vi "AlGaInPAs_v21a.vi"(2 "Debug Mode":bool, 3 "Elapsed Time(s)":dbl, 4 "State":enum16{"Edit", "Start", "Run", "End", "Idle"}(ring), 5 "Argument List In":string[](array[string])) -> (0 "Status Out":string, 1 "Argument List Out":string[](array[string]))   [LabVIEW 2011]
uses:
  high_level_proc/source_noDilute.ctl
  high_level_proc/source_noDilution.ctl
panel:
  in  "Zn bubbler":T1={"Dilution"=FALSE, "Calculated"=0, "MFC1 flow"=0.0, "MFC2 flow"=10.0, "MFC3 flow"=100.0, "Bubbler (main)"={"Flow"=0.0, "Prep"=FALSE, "Run"=FALSE, "Active"=FALSE}} caption="Al" {"Bubbler (main)"."Flow" format="%.2f"; "MFC1 flow" format="%.4f"; "MFC3 flow" format="%.1f"; "MFC2 flow" format="%.2f"; "Calculated" items=["Flow", "MFC1", "MFC2", "MFC3"]}
  in  "Array":refnum<vi>[](array[refnum])
  in  "Al bubbler":T2 caption="Al" {"Flow" format="%.2f"}
  in  "Se bubbler":T1={"Dilution"=FALSE, "Calculated"=0, "MFC1 flow"=0.0, "MFC2 flow"=10.0, "MFC3 flow"=100.0, "Bubbler (main)"={"Flow"=0.0, "Prep"=FALSE, "Run"=FALSE, "Active"=FALSE}} caption="Al" {"Bubbler (main)"."Flow" format="%.2f"; "MFC1 flow" format="%.4f"; "MFC3 flow" format="%.1f"; "MFC2 flow" format="%.2f"; "Calculated" items=["Flow", "MFC1", "MFC2", "MFC3"]}
  in  "P bubbler":T2 caption="Al" {"Flow" format="%.2f"}
  in  "As gas":T2 caption="Al" {"Flow" format="%.2f"}
  in  "P gas":T2 caption="Al" {"Flow" format="%.2f"}
  in  "In bubbler":T2 caption="Al" {"Flow" format="%.2f"}
  in  "Tab Control":T3(tab)
  out "Al Prep":bool caption="Pre-run"
  out "Al Run":bool caption="Run"
  out "Al Flow":dbl caption="Al Flow (0-100 sscm)" format="%.2f"
  out "Ga MFC1 flow":dbl caption="R1 (0-10 sscm)" format="%.4f"
  out "Ga MFC3 flow":dbl=100.0 caption="R3 (0-1000 sscm)" format="%.1f"
  out "Ga MFC2 flow":dbl=10.0 caption="R2 (0-100 sscm)" format="%.2f"
  out "Ga Calculated":u16(ring)=1 caption="Calculated" items=["Ga flow", "MFC1", "MFC2", "MFC3"]
  out "Ga Dilution":bool caption="Dilute"
  out "Ga Prep":bool caption="Pre-run"
  out "Ga Run":bool caption="Run"
  out "Ga Flow":dbl caption="Ga Flow (0-10 sscm)" format="%.2f"
  out "In Prep":bool caption="Pre-run"
  out "In Run":bool caption="Run"
  out "In Flow":dbl caption="In Flow (0-100 sscm)" format="%.2f"
  out "P gas Run":bool caption="Run"
  out "P gas Prep":bool caption="Pre-run"
  out "P gas Flow":dbl caption="PH3 Flow (0-100 sscm)" format="%.2f"
  out "As gas Prep":bool caption="Pre-run"
  out "As gas Run":bool caption="Run"
  out "As gas Flow":dbl caption="AsH3 Flow (0-10 sscm)" format="%.2f"
  out "P liq Prep":bool caption="Pre-run"
  out "P liq Run":bool caption="Run"
  out "P liq Flow":dbl caption="P bubbler Flow (0-100 sscm)" format="%.2f"
  out "Zn Flow":dbl caption="Zn Flow (0-10 sscm)" format="%.2f"
  out "Zn Run":bool caption="Run"
  out "Zn Prep":bool caption="Pre-run"
  out "Zn  Dilution":bool caption="Dilute"
  out "Zn Calculated":u16(ring)=1 caption="Calculated" items=["Ga flow", "MFC1", "MFC2", "MFC3"]
  out "Zn MFC2 flow":dbl=10.0 caption="R2 (0-100 sscm)" format="%.2f"
  out "Zn MFC3 flow":dbl=100.0 caption="R3 (0-1000 sscm)" format="%.1f"
  out "Zn MFC1 flow":dbl caption="R1 (0-10 sscm)" format="%.4f"
  out "Se MFC1 flow":dbl caption="R1 (0-10 sscm)" format="%.4f"
  out "Se MFC3 flow":dbl=100.0 caption="R3 (0-1000 sscm)" format="%.1f"
  out "Se MFC2 flow":dbl=10.0 caption="R2 (0-100 sscm)" format="%.2f"
  out "Se Calculated":u16(ring)=1 caption="Calculated" items=["Ga flow", "MFC1", "MFC2", "MFC3"]
  out "Se Dilution":bool caption="Dilute"
  out "Se Prep":bool caption="Pre-run"
  out "Se Run":bool caption="Run"
  out "Se Flow":dbl caption="Se Flow (0-10 sscm)" format="%.2f"
  in  "Ga bubbler":T1={"Dilution"=FALSE, "Calculated"=0, "MFC1 flow"=0.0, "MFC2 flow"=10.0, "MFC3 flow"=100.0, "Bubbler (main)"={"Flow"=0.0, "Prep"=FALSE, "Run"=FALSE, "Active"=FALSE}} caption="Al" {"Bubbler (main)"."Flow" format="%.2f"; "MFC1 flow" format="%.4f"; "MFC3 flow" format="%.1f"; "MFC2 flow" format="%.2f"; "Calculated" items=["Flow", "MFC1", "MFC2", "MFC3"]}
  out "prep_done":bool
  out "run started":bool
  out "first":bool=TRUE
  out "total time":dbl
  out "is OK?":bool
  in  "prep_time":dbl
  in  "Cancel":bool
  in  "OK":bool
  out "tTotal(s) 2":dbl
  # "s"
  # "Add pre-run time to run time in editor."
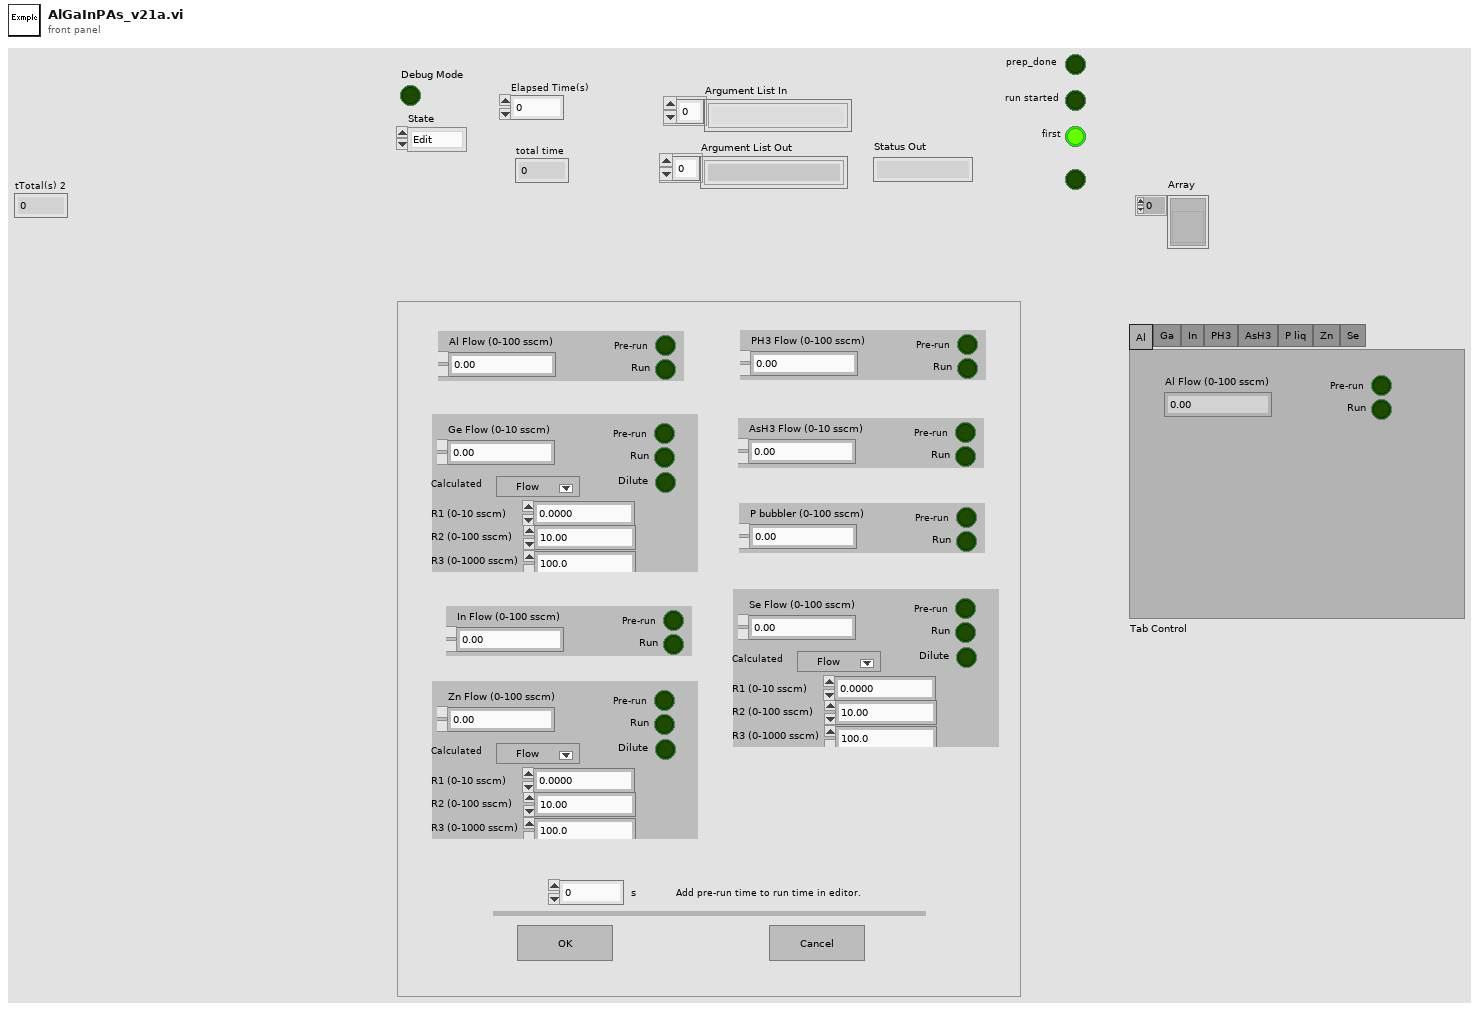
[diagram p1: front panel]
types:
  T1 = typedef "source_noDilute.ctl" = cluster{"Dilution":bool, "Calculated":u16, "MFC1 flow":dbl, "MFC2 flow":dbl, "MFC3 flow":dbl, "Bubbler (main)":T2}
  T2 = typedef "source_noDilution.ctl" = cluster{"Flow":dbl, "Prep":bool, "Run":bool, "Active":bool}
  T3 = enum32{"Al", "Ga", "In", "PH3", "AsH3", "P liq", "Zn", "Se"}
  T4 = enum16{"Discrete", "Continuous", "Instantaneous", "Finite"}
  T5 = enum32{"Invalid", "Default", "Floating", "Floating/Auto-Hide", "Modal"}
  T6 = cluster{"Flow":dbl, "Prep":bool, "Run":bool, "Active":bool}
  T7 = cluster{"Dilution":bool, "Calculated":u16, "MFC1 flow":dbl, "MFC2 flow":dbl, "MFC3 flow":dbl, "Bubbler (main)":T2}
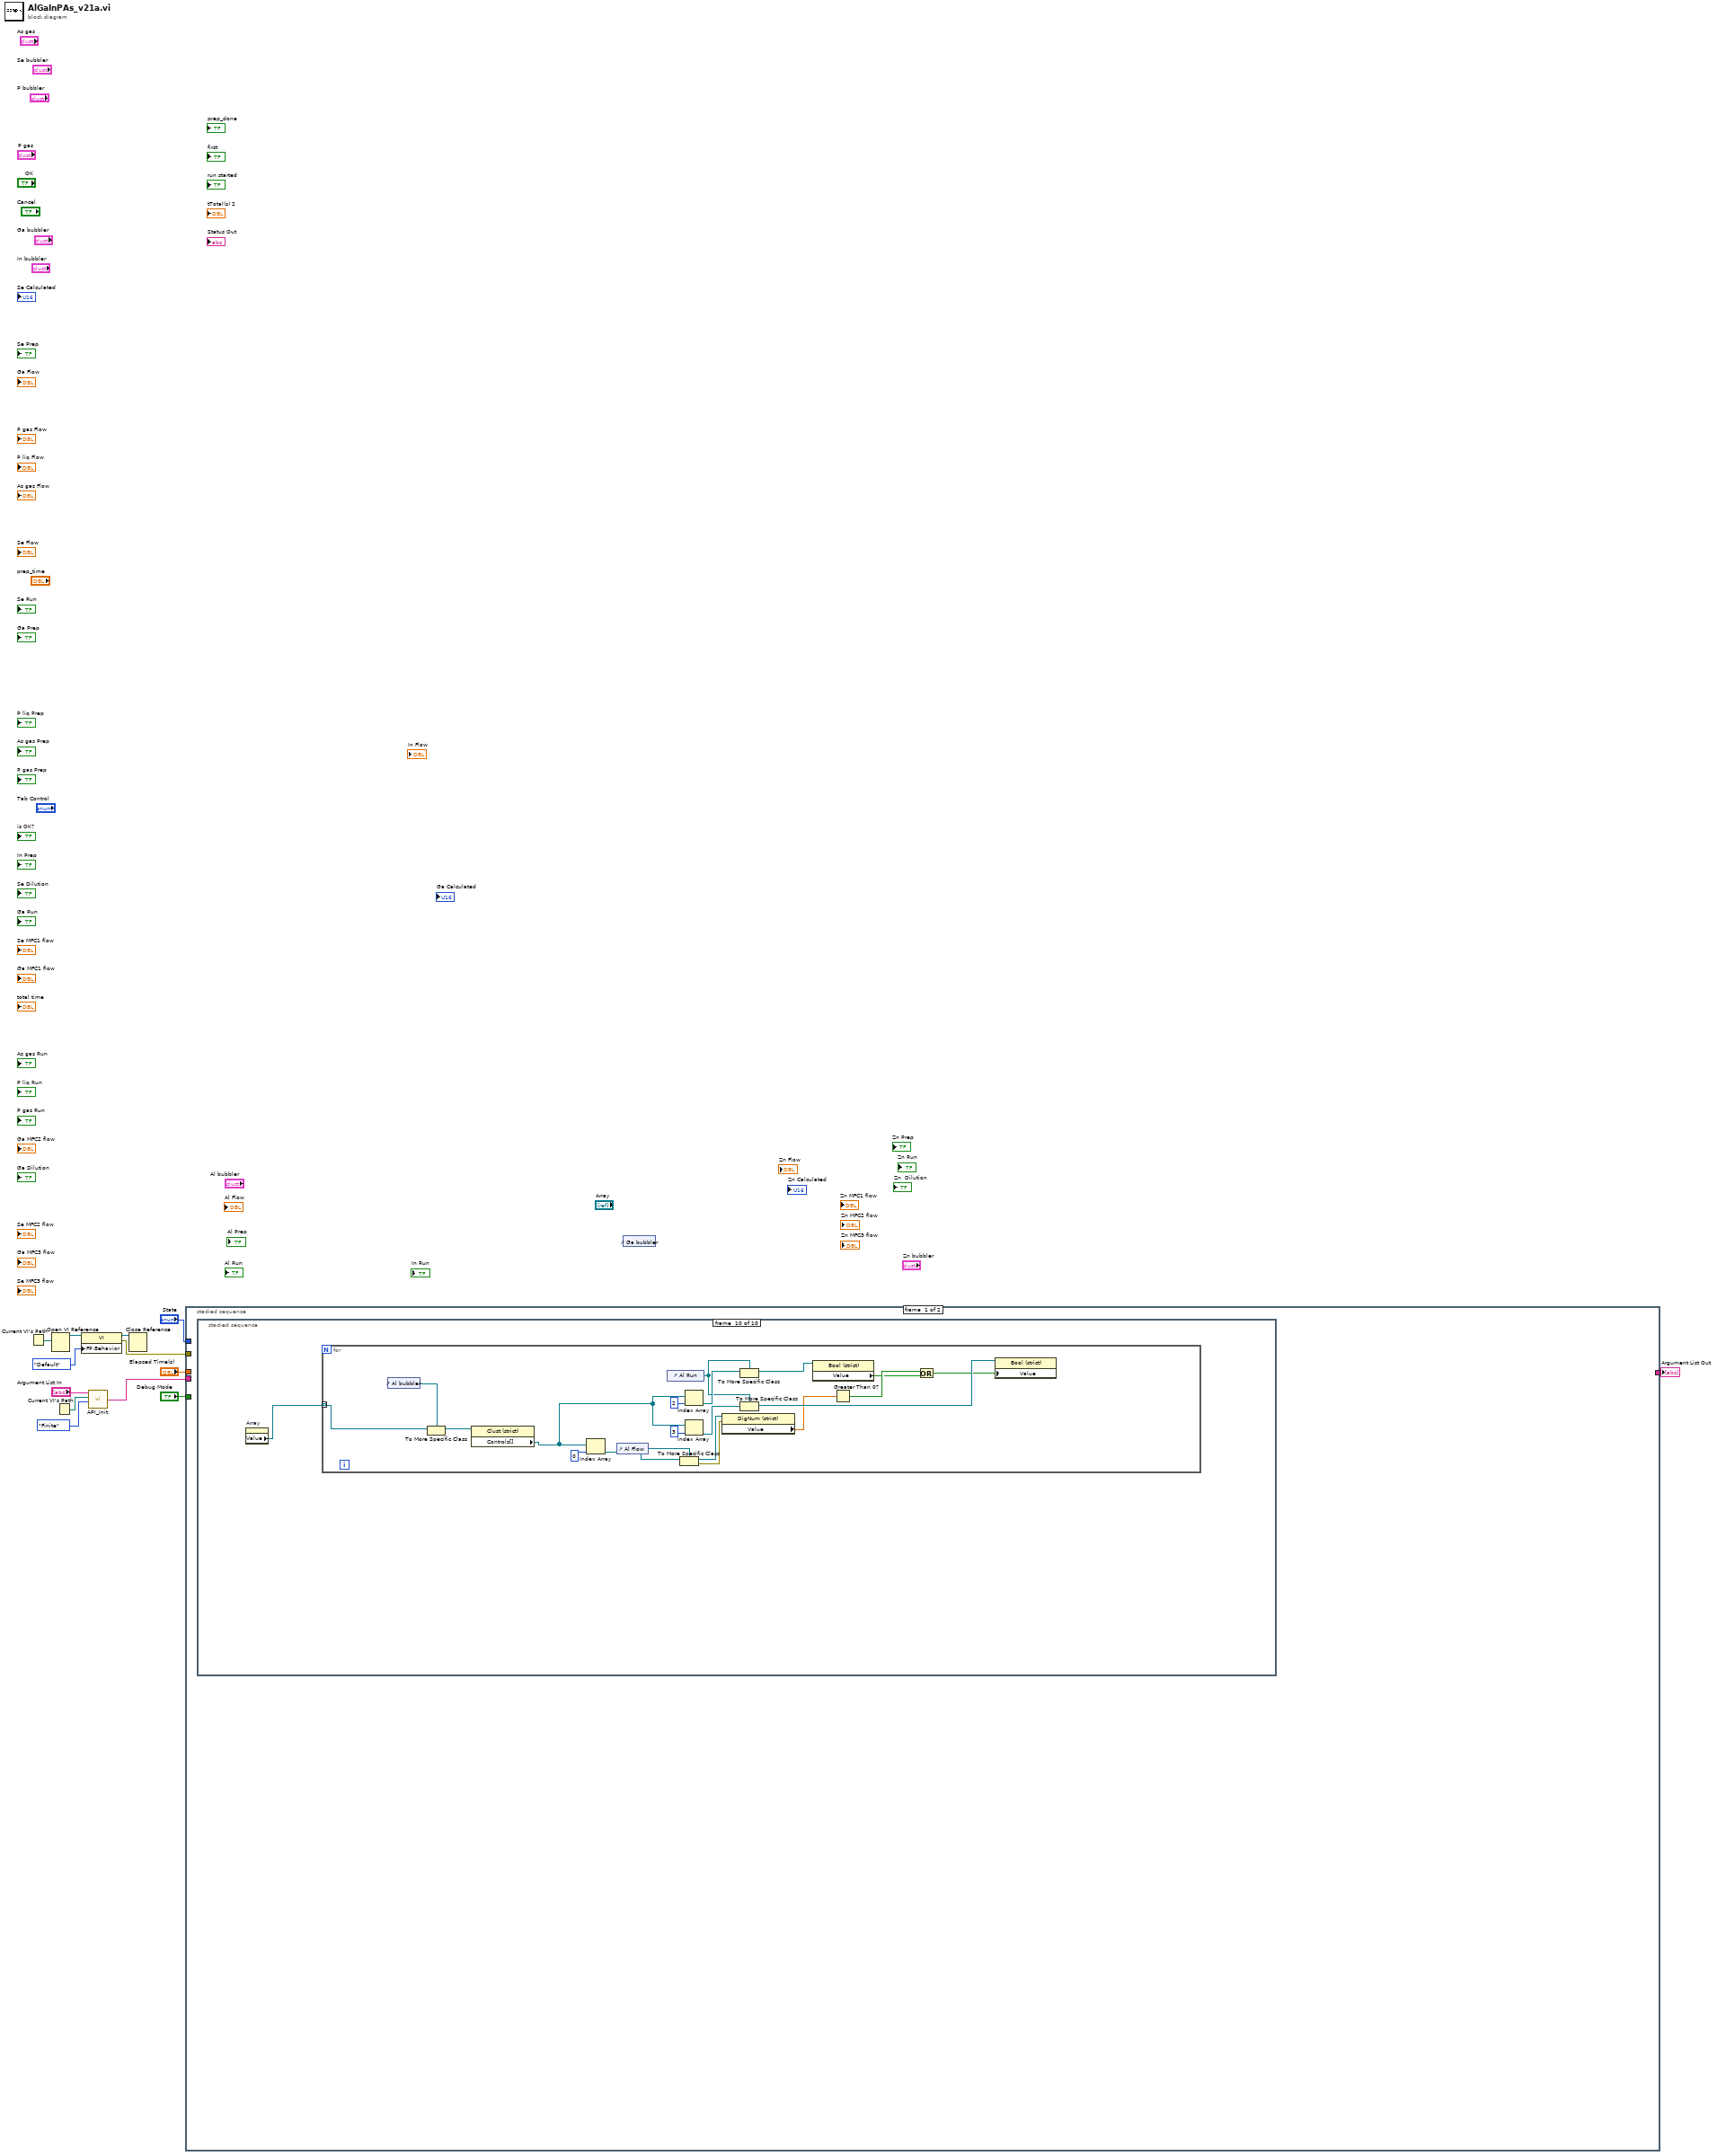
[diagram p0: block diagram]
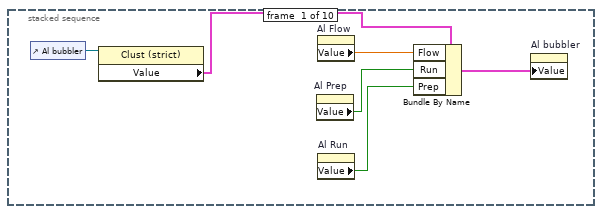
[diagram p2: hidden frame]
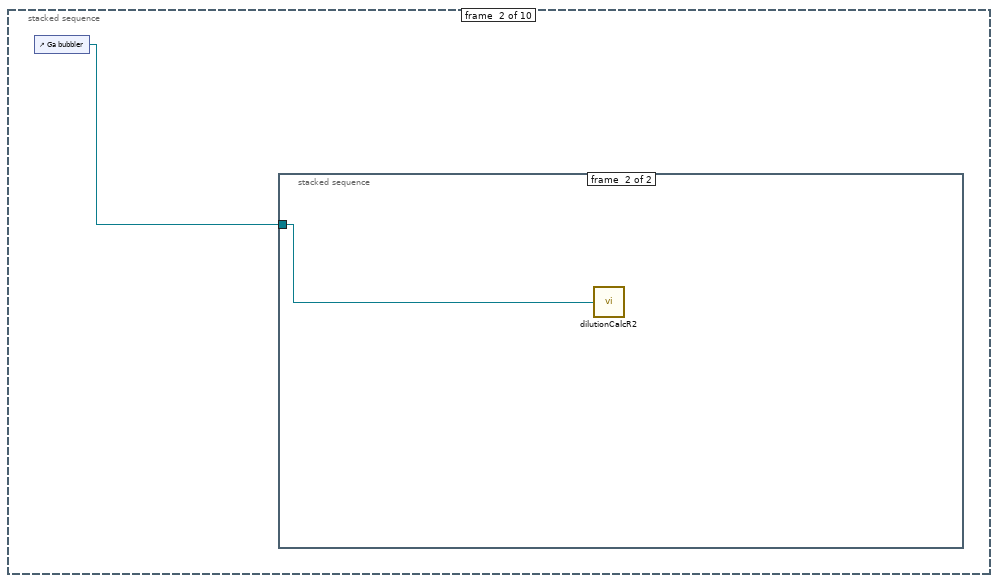
[diagram p3: hidden frame]
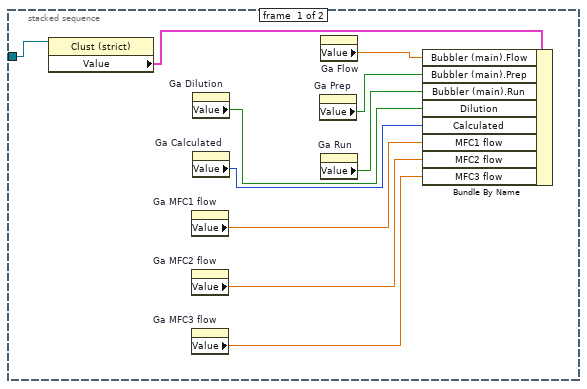
[diagram p4: hidden frame]
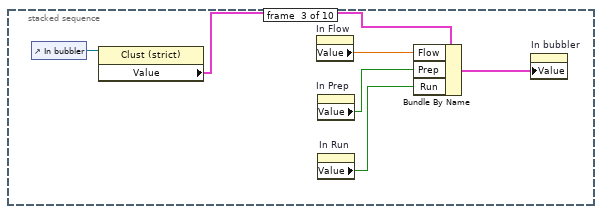
[diagram p5: hidden frame]
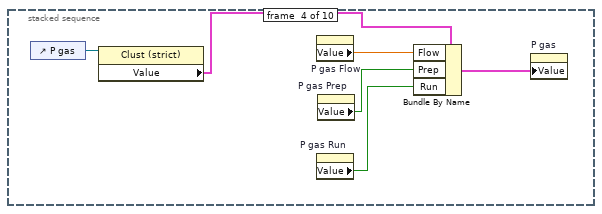
[diagram p6: hidden frame]
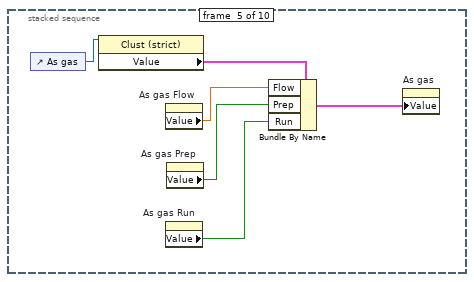
[diagram p7: hidden frame]
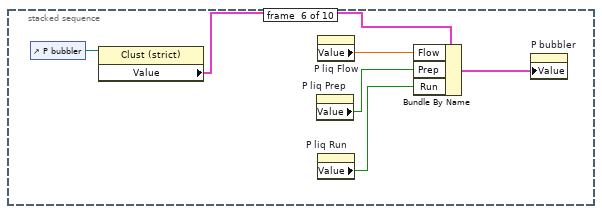
[diagram p8: hidden frame]
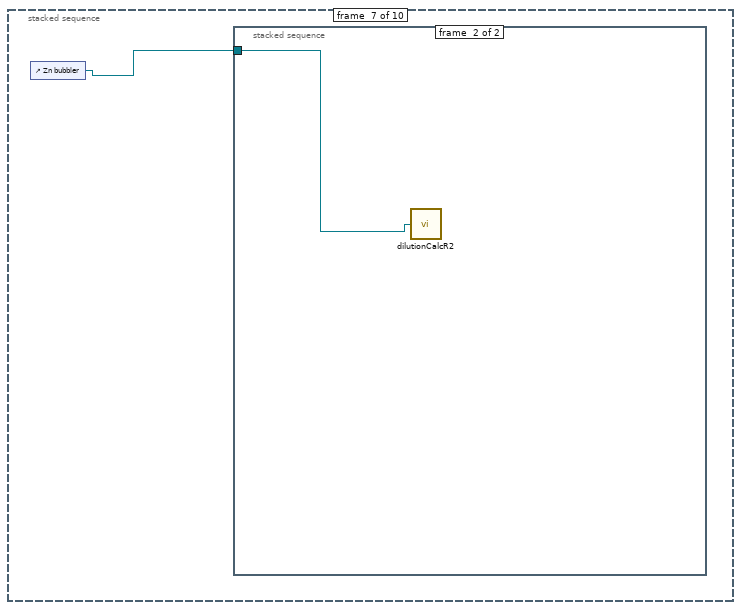
[diagram p9: hidden frame]
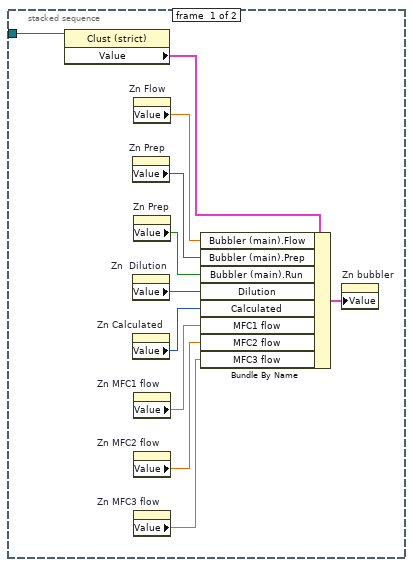
[diagram p10: hidden frame]
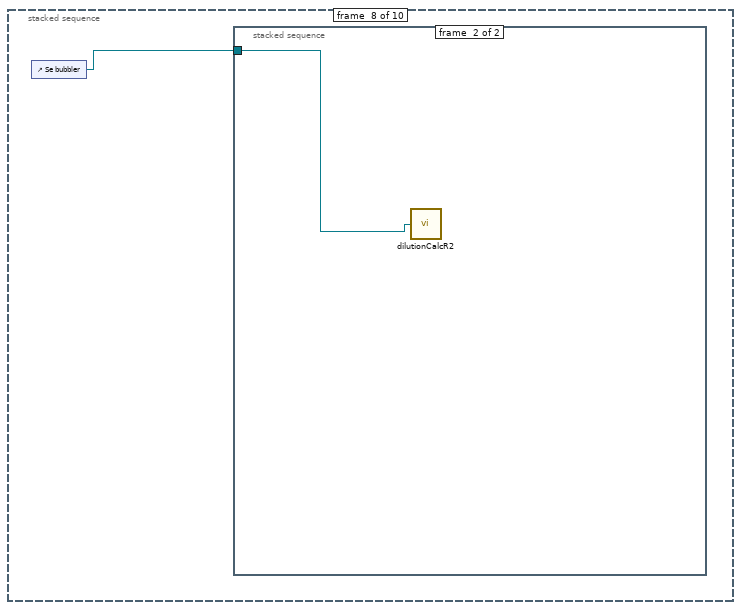
[diagram p11: hidden frame]
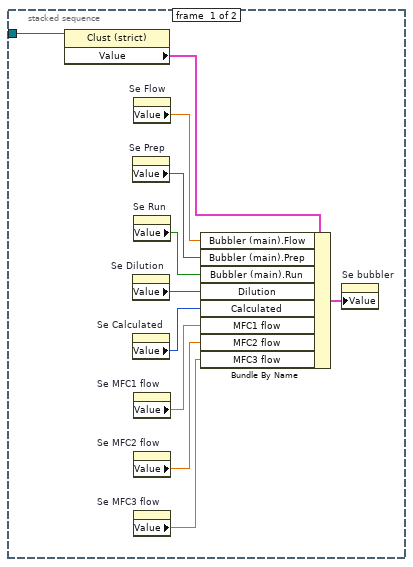
[diagram p12: hidden frame]
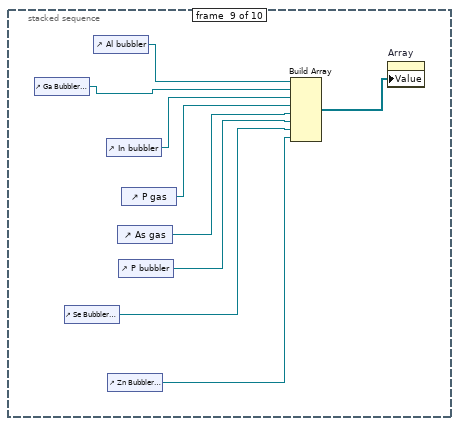
[diagram p13: hidden frame]
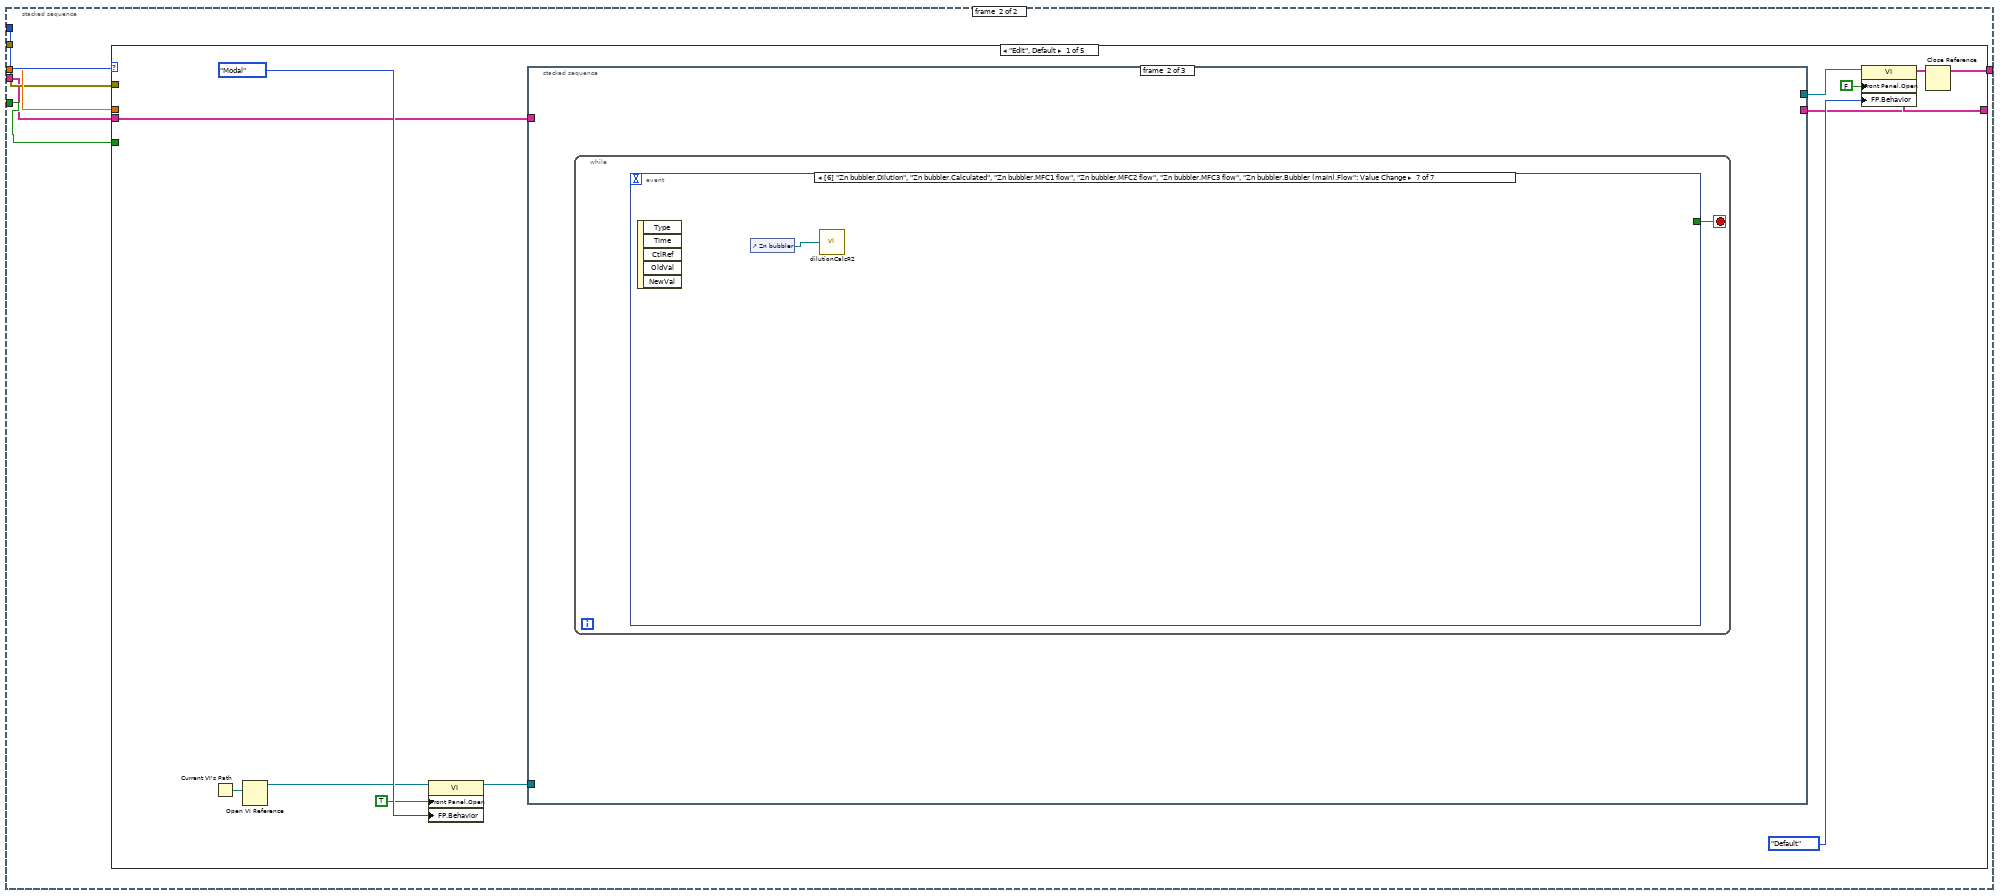
[diagram p14: hidden frame]
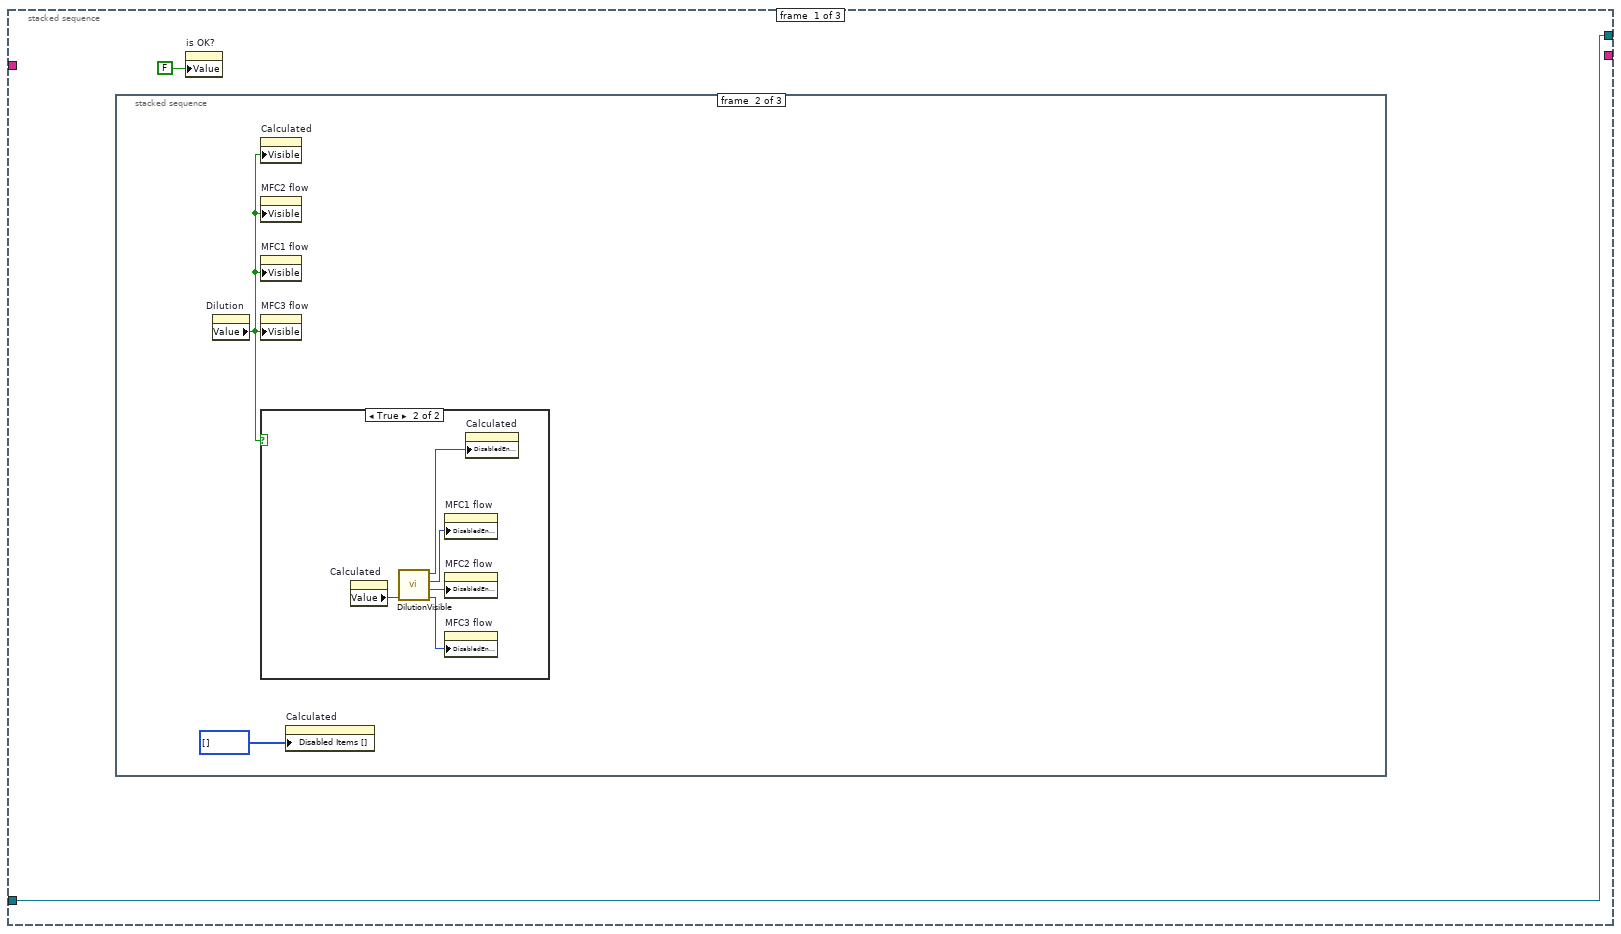
[diagram p15: hidden frame]
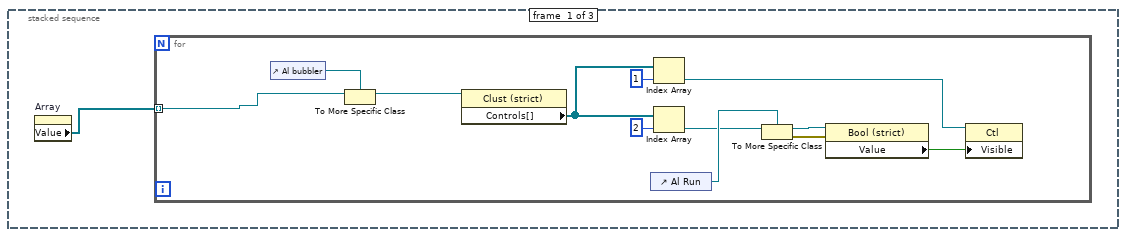
[diagram p16: hidden frame]
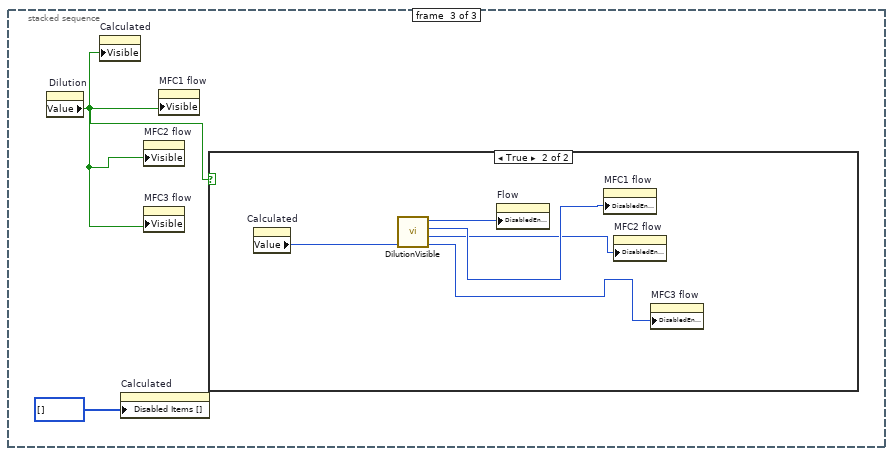
[diagram p18: hidden frame]
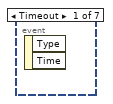
[diagram p20: hidden frame]
diagram:
  n1 = Current VI's Path() -> (path=w9:path)
  n2 = Open VI Reference(vi path=w9) -> (vi reference=w8:refnum<vi>)  [unwired: 1 in, 5 out]
  n3 = Current VI's Path() -> (path=w4:path)
  n4 = property class="VI"(reference=w8, "FP.Behavior"=T5."Default" ("Front Panel Window:Behavior")) -> (reference out=w6:refnum<vi>, error out=w5:errorcluster)  [unwired: 1 in]
  n5 = call "API_Init.vi"("API Mode"=T4."Finite", "VI Path"=w4, "Argument List In"="Argument List In") -> ("Argument List Out"=w1:string[])  [unwired: 1 in]
  n6 = Close Reference(reference=w6) -> ()  [unwired: 1 in, 1 out]
  n7 = stacked-sequence {
    tunnel: "State" -> [_ w117]
    tunnel: "Debug Mode" -> [_ w116]
    tunnel: "Elapsed Time(s)" -> [_ w115]
    tunnel: [_ w114] -> w10
    tunnel: w5 -> [_ w113]
    tunnel: w1 -> [_ w112]
    frame #0 {
      n8 = stacked-sequence {
        frame #0 {
          n9 = control-ref of="Al bubbler"() -> (w16:refnum<vi>)
          n10 = property class="Clust (strict)"(reference=w16) -> ("Value"=w15:T6)  [unwired: 1 in, 2 out]
          n11 = property on="Al Prep" class="Bool (strict)"() -> ("Value"=w18:bool)  [unwired: 2 in, 2 out]
          n12 = property on="Al Flow" class="DigNum (strict)"() -> ("Value"=w19:dbl)  [unwired: 2 in, 2 out]
          n13 = property on="Al Run" class="Bool (strict)"() -> ("Value"=w17:bool)  [unwired: 2 in, 2 out]
          n14 = Bundle By Name(cluster=w15, "Flow"=w19, "Run"=w18, "Prep"=w17) -> (w14:T6)
          n15 = property on="Al bubbler" class="Clust (strict)"("Value"=w14) -> ()  [unwired: 2 in, 2 out]
        }
        frame #1 {
          n16 = control-ref of="Ga bubbler"() -> (w20:refnum<vi>)
          n17 = stacked-sequence {
            tunnel: w20 -> [w22 w31]
            frame #0 {
              n18 = property class="Clust (strict)"(reference=w22) -> ("Value"=w21:T7)  [unwired: 1 in, 2 out]
              n19 = property on="Ga MFC1 flow" class="DigNum (strict)"() -> ("Value"=w28:dbl)  [unwired: 2 in, 2 out]
              n20 = property on="Ga MFC2 flow" class="DigNum (strict)"() -> ("Value"=w29:dbl)  [unwired: 2 in, 2 out]
              n21 = property on="Ga MFC3 flow" class="DigNum (strict)"() -> ("Value"=w30:dbl)  [unwired: 2 in, 2 out]
              n22 = property on="Ga Dilution" class="Bool (strict)"() -> ("Value"=w27:bool)  [unwired: 2 in, 2 out]
              n23 = property on="Ga Calculated" class="Ring (strict)"() -> ("Value"=w25:u16)  [unwired: 2 in, 2 out]
              n24 = property on="Ga Prep" class="Bool (strict)"() -> ("Value"=w24:bool)  [unwired: 2 in, 2 out]
              n25 = property on="Ga Flow" class="DigNum (strict)"() -> ("Value"=w23:dbl)  [unwired: 2 in, 2 out]
              n26 = property on="Ga Run" class="Bool (strict)"() -> ("Value"=w26:bool)  [unwired: 2 in, 2 out]
              n27 = Bundle By Name(cluster=w21, "Bubbler (main).Flow"=w23, "Bubbler (main).Prep"=w24, "Bubbler (main).Run"=w26, "Dilution"=w27, "Calculated"=w25, "MFC1 flow"=w28, "MFC2 flow"=w29, "MFC3 flow"=w30) -> ()  [unwired: 1 out]
            }
            frame #1 {
              n28 = call "dilutionCalcR2.vi"("Clust Refnum"=w31) -> ()
            }
          }
        }
        frame #2 {
          n29 = control-ref of="In bubbler"() -> (w32:refnum<vi>)
          n30 = property class="Clust (strict)"(reference=w32) -> ("Value"=w33:T6)  [unwired: 1 in, 2 out]
          n31 = property on="In Flow" class="DigNum (strict)"() -> ("Value"=w34:dbl)  [unwired: 2 in, 2 out]
          n32 = property on="In Prep" class="Bool (strict)"() -> ("Value"=w36:bool)  [unwired: 2 in, 2 out]
          n33 = property on="In Run" class="Bool (strict)"() -> ("Value"=w37:bool)  [unwired: 2 in, 2 out]
          n34 = Bundle By Name(cluster=w33, "Flow"=w34, "Prep"=w36, "Run"=w37) -> (w35:T6)
          n35 = property on="In bubbler" class="Clust (strict)"("Value"=w35) -> ()  [unwired: 2 in, 2 out]
        }
        frame #3 {
          n36 = control-ref of="P gas"() -> (w38:refnum<vi>)
          n37 = property class="Clust (strict)"(reference=w38) -> ("Value"=w39:T6)  [unwired: 1 in, 2 out]
          n38 = property on="P gas Flow" class="DigNum (strict)"() -> ("Value"=w40:dbl)  [unwired: 2 in, 2 out]
          n39 = property on="P gas Run" class="Bool (strict)"() -> ("Value"=w43:bool)  [unwired: 2 in, 2 out]
          n40 = property on="P gas Prep" class="Bool (strict)"() -> ("Value"=w42:bool)  [unwired: 2 in, 2 out]
          n41 = Bundle By Name(cluster=w39, "Flow"=w40, "Prep"=w42, "Run"=w43) -> (w41:T6)
          n42 = property on="P gas" class="Clust (strict)"("Value"=w41) -> ()  [unwired: 2 in, 2 out]
        }
        frame #4 {
          n43 = control-ref of="As gas"() -> (w45:refnum<vi>)
          n44 = property class="Clust (strict)"(reference=w45) -> ("Value"=w44:T6)  [unwired: 1 in, 2 out]
          n45 = property on="As gas Flow" class="DigNum (strict)"() -> ("Value"=w47:dbl)  [unwired: 2 in, 2 out]
          n46 = property on="As gas Run" class="Bool (strict)"() -> ("Value"=w49:bool)  [unwired: 2 in, 2 out]
          n47 = property on="As gas Prep" class="Bool (strict)"() -> ("Value"=w48:bool)  [unwired: 2 in, 2 out]
          n48 = Bundle By Name(cluster=w44, "Flow"=w47, "Prep"=w48, "Run"=w49) -> (w46:T6)
          n49 = property on="As gas" class="Clust (strict)"("Value"=w46) -> ()  [unwired: 2 in, 2 out]
        }
        frame #5 {
          n50 = control-ref of="P bubbler"() -> (w50:refnum<vi>)
          n51 = property class="Clust (strict)"(reference=w50) -> ("Value"=w51:T6)  [unwired: 1 in, 2 out]
          n52 = property on="P liq Prep" class="Bool (strict)"() -> ("Value"=w54:bool)  [unwired: 2 in, 2 out]
          n53 = property on="P liq Flow" class="DigNum (strict)"() -> ("Value"=w53:dbl)  [unwired: 2 in, 2 out]
          n54 = property on="P liq Run" class="Bool (strict)"() -> ("Value"=w55:bool)  [unwired: 2 in, 2 out]
          n55 = Bundle By Name(cluster=w51, "Flow"=w53, "Prep"=w54, "Run"=w55) -> (w52:T6)
          n56 = property on="P bubbler" class="Clust (strict)"("Value"=w52) -> ()  [unwired: 2 in, 2 out]
        }
        frame #6 {
          n57 = control-ref of="Zn bubbler"() -> (w56:refnum<vi>)
          n58 = stacked-sequence {
            tunnel: w56 -> [w57 w68]
            frame #0 {
              n59 = property class="Clust (strict)"(reference=w57) -> ("Value"=w58:T7)  [unwired: 1 in, 2 out]
              n60 = property on="Zn Prep" class="Bool (strict)"() -> ("Value"=w61:bool)  [unwired: 2 in, 2 out]
              n61 = property on="Zn  Dilution" class="Bool (strict)"() -> ("Value"=w63:bool)  [unwired: 2 in, 2 out]
              n62 = property on="Zn Calculated" class="Ring (strict)"() -> ("Value"=w64:u16)  [unwired: 2 in, 2 out]
              n63 = property on="Zn Flow" class="DigNum (strict)"() -> ("Value"=w60:dbl)  [unwired: 2 in, 2 out]
              n64 = property on="Zn Prep" class="Bool (strict)"() -> ("Value"=w62:bool)  [unwired: 2 in, 2 out]
              n65 = property on="Zn MFC1 flow" class="DigNum (strict)"() -> ("Value"=w65:dbl)  [unwired: 2 in, 2 out]
              n66 = property on="Zn MFC2 flow" class="DigNum (strict)"() -> ("Value"=w66:dbl)  [unwired: 2 in, 2 out]
              n67 = property on="Zn MFC3 flow" class="DigNum (strict)"() -> ("Value"=w67:dbl)  [unwired: 2 in, 2 out]
              n68 = Bundle By Name(cluster=w58, "Bubbler (main).Flow"=w60, "Bubbler (main).Prep"=w61, "Bubbler (main).Run"=w62, "Dilution"=w63, "Calculated"=w64, "MFC1 flow"=w65, "MFC2 flow"=w66, "MFC3 flow"=w67) -> (w59:T7)
              n69 = property on="Zn bubbler" class="Clust (strict)"("Value"=w59) -> ()  [unwired: 2 in, 2 out]
            }
            frame #1 {
              n70 = call "dilutionCalcR2.vi"("Clust Refnum"=w68) -> ()
            }
          }
        }
        frame #7 {
          n71 = control-ref of="Se bubbler"() -> (w69:refnum<vi>)
          n72 = stacked-sequence {
            tunnel: w69 -> [w70 w81]
            frame #0 {
              n73 = property class="Clust (strict)"(reference=w70) -> ("Value"=w71:T7)  [unwired: 1 in, 2 out]
              n74 = property on="Se Prep" class="Bool (strict)"() -> ("Value"=w74:bool)  [unwired: 2 in, 2 out]
              n75 = property on="Se Dilution" class="Bool (strict)"() -> ("Value"=w76:bool)  [unwired: 2 in, 2 out]
              n76 = property on="Se Calculated" class="Ring (strict)"() -> ("Value"=w77:u16)  [unwired: 2 in, 2 out]
              n77 = property on="Se Flow" class="DigNum (strict)"() -> ("Value"=w73:dbl)  [unwired: 2 in, 2 out]
              n78 = property on="Se Run" class="Bool (strict)"() -> ("Value"=w75:bool)  [unwired: 2 in, 2 out]
              n79 = property on="Se MFC1 flow" class="DigNum (strict)"() -> ("Value"=w78:dbl)  [unwired: 2 in, 2 out]
              n80 = property on="Se MFC2 flow" class="DigNum (strict)"() -> ("Value"=w79:dbl)  [unwired: 2 in, 2 out]
              n81 = property on="Se MFC3 flow" class="DigNum (strict)"() -> ("Value"=w80:dbl)  [unwired: 2 in, 2 out]
              n82 = Bundle By Name(cluster=w71, "Bubbler (main).Flow"=w73, "Bubbler (main).Prep"=w74, "Bubbler (main).Run"=w75, "Dilution"=w76, "Calculated"=w77, "MFC1 flow"=w78, "MFC2 flow"=w79, "MFC3 flow"=w80) -> (w72:T7)
              n83 = property on="Se bubbler" class="Clust (strict)"("Value"=w72) -> ()  [unwired: 2 in, 2 out]
            }
            frame #1 {
              n84 = call "dilutionCalcR2.vi"("Clust Refnum"=w81) -> ()
            }
          }
        }
        frame #8 {
          n85 = control-ref of="Ga Bubbler (main)"() -> (w84:refnum<vi>)
          n86 = control-ref of="Se Bubbler (main)"() -> (w83:refnum<vi>)
          n87 = control-ref of="Al bubbler"() -> (w89:refnum<vi>)
          n88 = control-ref of="In bubbler"() -> (w88:refnum<vi>)
          n89 = control-ref of="Zn Bubbler (main)"() -> (w82:refnum<vi>)
          n90 = control-ref of="As gas"() -> (w86:refnum<vi>)
          n91 = control-ref of="P bubbler"() -> (w85:refnum<vi>)
          n92 = control-ref of="P gas"() -> (w87:refnum<vi>)
          n93 = Build Array(w89, w84, w88, w87, w86, w85, w83, w82) -> (w90:refnum<vi>[])
          n94 = property on="Array" class="Arr (strict)"("Value"=w90) -> ()  [unwired: 2 in, 2 out]
        }
        frame #9 {
          n95 = property on="Array" class="Arr (strict)"() -> ("Value"=w91:refnum<vi>[])  [unwired: 2 in, 2 out]
          n96 = for {
            tunnel: w91 -> [w92] mode=indexing
            n97 = control-ref of="Al bubbler"() -> (w95:refnum<vi>)
            n98 = To More Specific Class(target class=w95, reference=w92) -> (specific class reference=w94:refnum<vi>)  [unwired: 1 in, 1 out]
            n99 = property class="Clust (strict)"(reference=w94) -> ("Controls[]"=w93:refnum<vi>[])  [unwired: 1 in, 2 out]
            n100 = Index Array(array=w93, index=0) -> (element=w107:refnum<vi>)
            n101 = control-ref of="Al Flow"() -> (w106:refnum<vi>)
            n102 = control-ref of="Al Run"() -> (w108:refnum<vi>)
            n103 = To More Specific Class(target class=w106, reference=w107) -> (specific class reference=w103:refnum<vi>, error out=w102:errorcluster)  [unwired: 1 in]
            n104 = Index Array(array=w93, index=2) -> (element=w110:refnum<vi>)
            n105 = Index Array(array=w93, index=3) -> (element=w109:refnum<vi>)
            n106 = property class="DigNum (strict)"(reference=w103, error in=w102) -> ("Value"=w101:dbl)  [unwired: 2 out]
            n107 = To More Specific Class(target class=w108, reference=w110) -> (specific class reference=w105:refnum<vi>)  [unwired: 1 in, 1 out]
            n108 = To More Specific Class(target class=w108, reference=w109) -> (specific class reference=w104:refnum<vi>)  [unwired: 1 in, 1 out]
            n109 = property class="Bool (strict)"(reference=w105) -> ("Value"=w100:bool)  [unwired: 1 in, 2 out]
            n110 = Greater Than 0?(x=w101) -> (x > 0?=w111:bool)
            n111 = Or(x=w111, y=w100) -> (x .or. y?=w99:bool)
            n112 = property class="Bool (strict)"(reference=w104, "Value"=w99) -> ()  [unwired: 1 in, 2 out]
          }
        }
      }
    }
    frame #1 {
      n113 = case shown="\"Edit\", Default" w117 {
        tunnel: w116 -> [_ w231 w250 _ _]
        tunnel: w115 -> [_ _ w251 _ _]
        tunnel: w112 -> [w119 w236 w249 w363 w364]
        tunnel: [w118 w235 w248 w363 w364] -> w114
        tunnel: w113 -> [_ _ _ _ _]
        frame "Edit", Default {
          n114 = Current VI's Path() -> (path=w124:path)
          n115 = Open VI Reference(vi path=w124) -> (vi reference=w123:refnum<vi>)  [unwired: 1 in, 5 out]
          n116 = property class="VI"(reference=w123, "Front Panel.Open"=TRUE ("Front Panel Window:Open"), "FP.Behavior"=T5."Modal" ("Front Panel Window:Behavior")) -> (reference out=w122:refnum<vi>)  [unwired: 1 in, 1 out]
          n117 = stacked-sequence {
            tunnel: w119 -> [_ _ w226]
            tunnel: w122 -> [w130 _ _]
            tunnel: [w130 _ _] -> w126
            tunnel: [_ _ w227] -> w118
            frame #0 {
              n118 = stacked-sequence {
                frame #0 {
                  n119 = property on="Array" class="Arr (strict)"() -> ("Value"=w131:refnum<vi>[])  [unwired: 2 in, 2 out]
                  n120 = for {
                    tunnel: w131 -> [w132] mode=indexing
                    n121 = control-ref of="Al bubbler"() -> (w133:refnum<vi>)
                    n122 = To More Specific Class(target class=w133, reference=w132) -> (specific class reference=w141:refnum<vi>)  [unwired: 1 in, 1 out]
                    n123 = property class="Clust (strict)"(reference=w141) -> ("Controls[]"=w140:refnum<vi>[])  [unwired: 1 in, 2 out]
                    n124 = control-ref of="Al Run"() -> (w138:refnum<vi>)
                    n125 = Index Array(array=w140, index=1) -> (element=w142:refnum<vi>)
                    n126 = Index Array(array=w140, index=2) -> (element=w137:refnum<vi>)
                    n127 = To More Specific Class(target class=w138, reference=w137) -> (specific class reference=w136:refnum<vi>, error out=w135:errorcluster)  [unwired: 1 in]
                    n128 = property class="Bool (strict)"(reference=w136, error in=w135) -> ("Value"=w134:bool)  [unwired: 2 out]
                    n129 = property class="Ctl"(reference=w142, "Visible"=w134) -> ()  [unwired: 1 in, 2 out]
                  }
                }
                frame #1 {
                  n130 = property on="Dilution" class="Bool (strict)"() -> ("Value"=w145:bool)  [unwired: 2 in, 2 out]
                  n131 = property on="Calculated" class="Ring (strict)"("Visible"=w145) -> ()  [unwired: 2 in, 2 out]
                  n132 = property on="MFC2 flow" class="DigNum (strict)"("Visible"=w145) -> ()  [unwired: 2 in, 2 out]
                  n133 = property on="MFC1 flow" class="DigNum (strict)"("Visible"=w145) -> ()  [unwired: 2 in, 2 out]
                  n134 = property on="MFC3 flow" class="DigNum (strict)"("Visible"=w145) -> ()  [unwired: 2 in, 2 out]
                  n135 = case shown="True" w145 {
                    frame False {
                    }
                    frame True {
                      n136 = property on="Calculated" class="Ring (strict)"() -> ("Value"=w147:u16)  [unwired: 2 in, 2 out]
                      n137 = call "DilutionVisible.vi"("calculated"=w147) -> ("MFC3"=w150:u16, "MFC2"=w149:u16, "MFC1"=w148:u16, "flow"=w146:u16)  [unwired: 3 in]
                      n138 = property on="MFC1 flow" class="DigNum (strict)"("DisabledEnum"=w148) -> ()  [unwired: 2 in, 2 out]
                      n139 = property on="MFC2 flow" class="DigNum (strict)"("DisabledEnum"=w149) -> ()  [unwired: 2 in, 2 out]
                      n140 = property on="MFC3 flow" class="DigNum (strict)"("DisabledEnum"=w150) -> ()  [unwired: 2 in, 2 out]
                      n141 = property on="Calculated" class="Ring (strict)"("DisabledEnum"=w146) -> ()  [unwired: 2 in, 2 out]
                    }
                  }
                  n142 = property on="Calculated" class="Ring (strict)"("Disabled Items []"=i32[] []) -> ()  [unwired: 2 in, 2 out]
                }
                frame #2 {
                  n143 = property on="Dilution" class="Bool (strict)"() -> ("Value"=w151:bool)  [unwired: 2 in, 2 out]
                  n144 = property on="Calculated" class="Ring (strict)"("Visible"=w151) -> ()  [unwired: 2 in, 2 out]
                  n145 = property on="Calculated" class="Ring (strict)"("Disabled Items []"=i32[] []) -> ()  [unwired: 2 in, 2 out]
                  n146 = property on="MFC2 flow" class="DigNum (strict)"("Visible"=w151) -> ()  [unwired: 2 in, 2 out]
                  n147 = property on="MFC3 flow" class="DigNum (strict)"("Visible"=w151) -> ()  [unwired: 2 in, 2 out]
                  n148 = property on="MFC1 flow" class="DigNum (strict)"("Visible"=w151) -> ()  [unwired: 2 in, 2 out]
                  n149 = case shown="True" w151 {
                    frame False {
                    }
                    frame True {
                      n150 = property on="Calculated" class="Ring (strict)"() -> ("Value"=w156:u16)  [unwired: 2 in, 2 out]
                      n151 = call "DilutionVisible.vi"("calculated"=w156) -> ("MFC3"=w154:u16, "MFC2"=w153:u16, "MFC1"=w155:u16, "flow"=w157:u16)  [unwired: 3 in]
                      n152 = property on="Flow" class="DigNum (strict)"("DisabledEnum"=w157) -> ()  [unwired: 2 in, 2 out]
                      n153 = property on="MFC1 flow" class="DigNum (strict)"("DisabledEnum"=w155) -> ()  [unwired: 2 in, 2 out]
                      n154 = property on="MFC2 flow" class="DigNum (strict)"("DisabledEnum"=w153) -> ()  [unwired: 2 in, 2 out]
                      n155 = property on="MFC3 flow" class="DigNum (strict)"("DisabledEnum"=w154) -> ()  [unwired: 2 in, 2 out]
                    }
                  }
                }
              }
              n156 = property on="is OK?" class="Bool (strict)"("Value"=FALSE ("is OK?")) -> ()  [unwired: 2 in, 2 out]
            }
            frame #1 {
              n157 = while {
                stop <- w158 stop-if-true
                n158 = event shown="[6] \"Zn bubbler.Dilution\", \"Zn bubbler.Calculated\", \"Zn bubbler.MFC1 flow\", \"Zn bubbler.MFC2 flow\", \"Zn bubbler.MFC3 flow\", \"Zn bubbler.Bubbler (main).Flow\": Value Change" {
                  selector: _ -> [_ _ _ _ _ _ _]
                  dyn-events: _ -> [_ _ _ _ _ _ _]
                  timeout: _ -> [_ _ _ _ _ _ _]
                  tunnel: [_ TRUE _ TRUE _ _ _] -> w158
                  event Timeout {
                    n159 = event-data() -> ()  [unwired: 1 in, 2 out]
                  }
                  event "OK": Value Change {
                    n160 = event-data() -> ()  [unwired: 1 in, 5 out]
                    n161 = stacked-sequence {
                      frame #0 {
                        n162 = property on="Al bubbler" class="Clust (strict)"() -> ("Value"=w161:T6)  [unwired: 2 in, 2 out]
                        n163 = Unbundle By Name(w161) -> ("Prep"=w164:bool, "Run"=w163:bool, "Flow"=w162:dbl)
                        n164 = property on="Al Prep" class="Bool (strict)"("Value"=w164) -> ()  [unwired: 2 in, 2 out]
                        n165 = property on="Al Run" class="Bool (strict)"("Value"=w163) -> ()  [unwired: 2 in, 2 out]
                        n166 = property on="Al Flow" class="DigNum (strict)"("Value"=w162) -> ()  [unwired: 2 in, 2 out]
                      }
                      frame #1 {
                        n167 = property on="Ga bubbler" class="Clust (strict)"() -> ("Value"=w173:T7)  [unwired: 2 in, 2 out]
                        n168 = Unbundle By Name(w173) -> ("Bubbler (main).Prep"=w172:bool, "Bubbler (main).Run"=w171:bool, "Bubbler (main).Flow"=w170:dbl, "Dilution"=w169:bool, "Calculated"=w168:u16, "MFC1 flow"=w167:dbl, "MFC2 flow"=w166:dbl, "MFC3 flow"=w165:dbl)
                        n169 = property on="Ga Prep" class="Bool (strict)"("Value"=w172) -> ()  [unwired: 2 in, 2 out]
                        n170 = property on="Ga Run" class="Bool (strict)"("Value"=w171) -> ()  [unwired: 2 in, 2 out]
                        n171 = property on="Ga Flow" class="DigNum (strict)"("Value"=w170) -> ()  [unwired: 2 in, 2 out]
                        n172 = property on="Ga Dilution" class="Bool (strict)"("Value"=w169) -> ()  [unwired: 2 in, 2 out]
                        n173 = property on="Ga Calculated" class="Ring (strict)"("Value"=w168) -> ()  [unwired: 2 in, 2 out]
                        n174 = property on="Ga MFC1 flow" class="DigNum (strict)"("Value"=w167) -> ()  [unwired: 2 in, 2 out]
                        n175 = property on="Ga MFC2 flow" class="DigNum (strict)"("Value"=w166) -> ()  [unwired: 2 in, 2 out]
                        n176 = property on="Ga MFC3 flow" class="DigNum (strict)"("Value"=w165) -> ()  [unwired: 2 in, 2 out]
                      }
                      frame #2 {
                        n177 = property on="In bubbler" class="Clust (strict)"() -> ("Value"=w177:T6)  [unwired: 2 in, 2 out]
                        n178 = Unbundle By Name(w177) -> ("Prep"=w176:bool, "Run"=w175:bool, "Flow"=w174:dbl)
                        n179 = property on="In Prep" class="Bool (strict)"("Value"=w176) -> ()  [unwired: 2 in, 2 out]
                        n180 = property on="In Run" class="Bool (strict)"("Value"=w175) -> ()  [unwired: 2 in, 2 out]
                        n181 = property on="In Flow" class="DigNum (strict)"("Value"=w174) -> ()  [unwired: 2 in, 2 out]
                      }
                      frame #3 {
                        n182 = property on="P gas" class="Clust (strict)"() -> ("Value"=w181:T6)  [unwired: 2 in, 2 out]
                        n183 = Unbundle By Name(w181) -> ("Prep"=w180:bool, "Run"=w179:bool, "Flow"=w178:dbl)
                        n184 = property on="P gas Prep" class="Bool (strict)"("Value"=w180) -> ()  [unwired: 2 in, 2 out]
                        n185 = property on="P gas Run" class="Bool (strict)"("Value"=w179) -> ()  [unwired: 2 in, 2 out]
                        n186 = property on="P gas Flow" class="DigNum (strict)"("Value"=w178) -> ()  [unwired: 2 in, 2 out]
                      }
                      frame #4 {
                        n187 = property on="As gas" class="Clust (strict)"() -> ("Value"=w185:T6)  [unwired: 2 in, 2 out]
                        n188 = Unbundle By Name(w185) -> ("Prep"=w184:bool, "Run"=w183:bool, "Flow"=w182:dbl)
                        n189 = property on="As gas Prep" class="Bool (strict)"("Value"=w184) -> ()  [unwired: 2 in, 2 out]
                        n190 = property on="As gas Run" class="Bool (strict)"("Value"=w183) -> ()  [unwired: 2 in, 2 out]
                        n191 = property on="As gas Flow" class="DigNum (strict)"("Value"=w182) -> ()  [unwired: 2 in, 2 out]
                      }
                      frame #5 {
                        n192 = property on="P bubbler" class="Clust (strict)"() -> ("Value"=w189:T6)  [unwired: 2 in, 2 out]
                        n193 = Unbundle By Name(w189) -> ("Prep"=w188:bool, "Run"=w187:bool, "Flow"=w186:dbl)
                        n194 = property on="P liq Prep" class="Bool (strict)"("Value"=w188) -> ()  [unwired: 2 in, 2 out]
                        n195 = property on="P liq Run" class="Bool (strict)"("Value"=w187) -> ()  [unwired: 2 in, 2 out]
                        n196 = property on="P liq Flow" class="DigNum (strict)"("Value"=w186) -> ()  [unwired: 2 in, 2 out]
                      }
                      frame #6 {
                        n197 = property on="Zn bubbler" class="Clust (strict)"() -> ("Value"=w198:T7)  [unwired: 2 in, 2 out]
                        n198 = Unbundle By Name(w198) -> ("Bubbler (main).Prep"=w197:bool, "Bubbler (main).Run"=w196:bool, "Bubbler (main).Flow"=w195:dbl, "Dilution"=w194:bool, "Calculated"=w193:u16, "MFC1 flow"=w192:dbl, "MFC2 flow"=w191:dbl, "MFC3 flow"=w190:dbl)
                        n199 = property on="Zn Prep" class="Bool (strict)"("Value"=w197) -> ()  [unwired: 2 in, 2 out]
                        n200 = property on="Zn Run" class="Bool (strict)"("Value"=w196) -> ()  [unwired: 2 in, 2 out]
                        n201 = property on="Zn Flow" class="DigNum (strict)"("Value"=w195) -> ()  [unwired: 2 in, 2 out]
                        n202 = property on="Zn  Dilution" class="Bool (strict)"("Value"=w194) -> ()  [unwired: 2 in, 2 out]
                        n203 = property on="Zn Calculated" class="Ring (strict)"("Value"=w193) -> ()  [unwired: 2 in, 2 out]
                        n204 = property on="Zn MFC1 flow" class="DigNum (strict)"("Value"=w192) -> ()  [unwired: 2 in, 2 out]
                        n205 = property on="Zn MFC2 flow" class="DigNum (strict)"("Value"=w191) -> ()  [unwired: 2 in, 2 out]
                        n206 = property on="Zn MFC3 flow" class="DigNum (strict)"("Value"=w190) -> ()  [unwired: 2 in, 2 out]
                      }
                      frame #7 {
                        n207 = property on="Se bubbler" class="Clust (strict)"() -> ("Value"=w207:T7)  [unwired: 2 in, 2 out]
                        n208 = Unbundle By Name(w207) -> ("Bubbler (main).Prep"=w206:bool, "Bubbler (main).Run"=w205:bool, "Bubbler (main).Flow"=w204:dbl, "Dilution"=w203:bool, "Calculated"=w202:u16, "MFC1 flow"=w201:dbl, "MFC2 flow"=w200:dbl, "MFC3 flow"=w199:dbl)
                        n209 = property on="Se Prep" class="Bool (strict)"("Value"=w206) -> ()  [unwired: 2 in, 2 out]
                        n210 = property on="Se Run" class="Bool (strict)"("Value"=w205) -> ()  [unwired: 2 in, 2 out]
                        n211 = property on="Se Flow" class="DigNum (strict)"("Value"=w204) -> ()  [unwired: 2 in, 2 out]
                        n212 = property on="Se Dilution" class="Bool (strict)"("Value"=w203) -> ()  [unwired: 2 in, 2 out]
                        n213 = property on="Se Calculated" class="Ring (strict)"("Value"=w202) -> ()  [unwired: 2 in, 2 out]
                        n214 = property on="Se MFC1 flow" class="DigNum (strict)"("Value"=w201) -> ()  [unwired: 2 in, 2 out]
                        n215 = property on="Se MFC2 flow" class="DigNum (strict)"("Value"=w200) -> ()  [unwired: 2 in, 2 out]
                        n216 = property on="Se MFC3 flow" class="DigNum (strict)"("Value"=w199) -> ()  [unwired: 2 in, 2 out]
                      }
                    }
                    n217 = property on="is OK?" class="Bool (strict)"("Value"=TRUE ("is OK?")) -> ()  [unwired: 2 in, 2 out]
                  }
                  event Value Change {
                    n218 = event-data() -> ()  [unwired: 1 in, 5 out]
                    n219 = property on="Array" class="Arr (strict)"() -> ("Value"=w208:refnum<vi>[])  [unwired: 2 in, 2 out]
                    n220 = for {
                      tunnel: w208 -> [w210] mode=indexing
                      n221 = control-ref of="Al bubbler"() -> (w209:refnum<vi>)
                      n222 = To More Specific Class(target class=w209, reference=w210) -> (specific class reference=w218:refnum<vi>)  [unwired: 1 in, 1 out]
                      n223 = property class="Clust (strict)"(reference=w218) -> ("Controls[]"=w217:refnum<vi>[])  [unwired: 1 in, 2 out]
                      n224 = control-ref of="Al Run"() -> (w211:refnum<vi>)
                      n225 = Index Array(array=w217, index=1) -> (element=w219:refnum<vi>)
                      n226 = Index Array(array=w217, index=2) -> (element=w215:refnum<vi>)
                      n227 = To More Specific Class(target class=w211, reference=w215) -> (specific class reference=w214:refnum<vi>, error out=w213:errorcluster)  [unwired: 1 in]
                      n228 = property class="Bool (strict)"(reference=w214, error in=w213) -> ("Value"=w212:bool)  [unwired: 2 out]
                      n229 = property class="Ctl"(reference=w219, "Visible"=w212) -> ()  [unwired: 1 in, 2 out]
                    }
                  }
                  event "Cancel": Value Change {
                    n230 = event-data() -> ()  [unwired: 1 in, 5 out]
                  }
                  event Value Change {
                    n231 = event-data() -> ()  [unwired: 1 in, 5 out]
                    n232 = control-ref of="Ga bubbler"() -> (w222:refnum<vi>)
                    n233 = call "dilutionCalcR2.vi"("Clust Refnum"=w222) -> ()
                  }
                  event Value Change {
                    n234 = event-data() -> ()  [unwired: 1 in, 5 out]
                    n235 = control-ref of="Se bubbler"() -> (w223:refnum<vi>)
                    n236 = call "dilutionCalcR2.vi"("Clust Refnum"=w223) -> ()
                  }
                  event Value Change {
                    n237 = event-data() -> ()  [unwired: 1 in, 5 out]
                    n238 = control-ref of="Zn bubbler"() -> (w224:refnum<vi>)
                    n239 = call "dilutionCalcR2.vi"("Clust Refnum"=w224) -> ()
                  }
                }
              }
            }
            frame #2 {
              n240 = property on="is OK?" class="Bool (strict)"() -> ("Value"=w225:bool)  [unwired: 2 in, 2 out]
              n241 = Not(x=w225) -> (.not. x?=w229:bool)
              n242 = Current VI's Path() -> (path=w228:path)
              n243 = call "API_Edit.vi"("Cancel"=w229, "OK"=w225, "VI Path"=w228, "Argument List In"=w226) -> ("Argument List Out"=w227:string[])
            }
          }
          n244 = property class="VI"(reference=w126, "Front Panel.Open"=FALSE ("Front Panel Window:Open"), "FP.Behavior"=T5."Default" ("Front Panel Window:Behavior")) -> (reference out=w127:refnum<vi>)  [unwired: 1 in, 1 out]
          n245 = Close Reference(reference=w127) -> ()  [unwired: 1 in, 1 out]
        }
        frame "Start" {
          n246 = property on="prep_time" class="DigNum (strict)"() -> ("Value"=w234:dbl)  [unwired: 2 in, 2 out]
          n247 = Greater Than 0?(x=w234) -> (x > 0?=w233:bool)
          n248 = Not(x=w231) -> (.not. x?=w230:bool)
          n249 = And(x=w230, y=w233) -> (x .and. y?=w232:bool)
          n250 = case shown="True" w232 {
            frame False {
            }
            frame True {
              n251 = property on="Ga bubbler" class="Clust (strict)"() -> ("Value"=w245:T7)  [unwired: 2 in, 2 out]
              n252 = property on="Zn bubbler" class="Clust (strict)"() -> ("Value"=w239:T7)  [unwired: 2 in, 2 out]
              n253 = property on="Al bubbler" class="Clust (strict)"() -> ("Value"=w246:T6)  [unwired: 2 in, 2 out]
              n254 = property on="In bubbler" class="Clust (strict)"() -> ("Value"=w244:T6)  [unwired: 2 in, 2 out]
              n255 = property on="P gas" class="Clust (strict)"() -> ("Value"=w243:T6)  [unwired: 2 in, 2 out]
              n256 = property on="Se bubbler" class="Clust (strict)"() -> ("Value"=w240:T7)  [unwired: 2 in, 2 out]
              n257 = property on="As gas" class="Clust (strict)"() -> ("Value"=w242:T6)  [unwired: 2 in, 2 out]
              n258 = property on="P bubbler" class="Clust (strict)"() -> ("Value"=w241:T6)  [unwired: 2 in, 2 out]
              n259 = call "Set_V_III.vi"("Se bubbler"=w240, "P bubbler"=w241, "As gas"=w242, "P gas"=w243, "Run Started"=FALSE, "Zn bubbler"=w239, "In bubbler"=w244, "Ga bubbler"=w245, "Al bubbler"=w246) -> ()  [unwired: 3 in]
            }
          }
          n260 = call "Set_Argument.vi"("Enable"=FALSE, "Argument"="run_started", "Argument List In"=w236) -> ("Argument List Out"=w235:string[])
        }
        frame "Run" {
          n261 = stacked-sequence {
            tunnel: w251 -> [_ w256 _ _]
            tunnel: w249 -> [w253 _ _ w339]
            tunnel: w250 -> [_ _ _ w337]
            tunnel: [_ _ _ w338] -> w248
            frame #0 {
              n262 = call "Get_Argument.vi"("Argument"="run_started", "Argument List"=w253) -> ("Enabled"=w252:bool)
              n263 = local write "run started"(w252) -> ()
            }
            frame #1 {
              n264 = property on="prep_time" class="DigNum (strict)"() -> ("Value"=w257:dbl)  [unwired: 2 in, 2 out]
              n265 = Greater Or Equal?(x=w256, y=w257) -> (x >= y?=w255:bool)
              n266 = local write "prep_done"(w255) -> ()
            }
            frame #2 {
              n267 = local read "run started"() -> (w259:bool)
              n268 = Not(x=w259) -> (.not. x?=w258:bool)
              n269 = stacked-sequence {
                tunnel: w258 -> [w261 w267 w276 w285 w294 w303 w312 w321 w330]
                frame #0 {
                  n270 = case shown="True" w261 {
                    tunnel: ["run: " "pre-run: "] -> w260
                    frame False {
                    }
                    frame True {
                    }
                  }
                  n271 = property on="Status Out" class="Str"("Value"=w260) -> ()  [unwired: 2 in, 2 out]
                }
                frame #1 {
                  n272 = property on="Al bubbler" class="Clust (strict)"() -> ("Value"=w264:T6)  [unwired: 2 in, 2 out]
                  n273 = Unbundle By Name(w264) -> ("Run"=w266:bool, "Prep"=w265:bool)
                  n274 = property on="Status Out" class="Str"() -> ("Value"=w272:string)  [unwired: 2 in, 2 out]
                  n275 = call "flow_strings.vi"("string in"=w272, "is first in?"=TRUE, "name"="Al", "run source?"=w266, "prep source?"=w265, "is prep?"=w267) -> ("string out"=w271:string, "is first out?"=w270:bool)  [unwired: 1 in]
                  n276 = property on="Status Out" class="Str"("Value"=w271) -> ()  [unwired: 2 in, 2 out]
                  n277 = property on="first" class="Bool (strict)"("Value"=w270) -> ()  [unwired: 2 in, 2 out]
                }
                frame #2 {
                  n278 = property on="Ga bubbler" class="Clust (strict)"() -> ("Value"=w275:T7)  [unwired: 2 in, 2 out]
                  n279 = Unbundle By Name(w275) -> ("Bubbler (main).Run"=w274:bool, "Bubbler (main).Prep"=w273:bool)
                  n280 = property on="Status Out" class="Str"() -> ("Value"=w280:string)  [unwired: 2 in, 2 out]
                  n281 = property on="first" class="Bool (strict)"() -> ("Value"=w278:bool)  [unwired: 2 in, 2 out]
                  n282 = call "flow_strings.vi"("string in"=w280, "is first in?"=w278, "name"="Ga", "run source?"=w274, "prep source?"=w273, "is prep?"=w276) -> ("string out"=w281:string, "is first out?"=w277:bool)  [unwired: 1 in]
                  n283 = property on="Status Out" class="Str"("Value"=w281) -> ()  [unwired: 2 in, 2 out]
                  n284 = property on="first" class="Bool (strict)"("Value"=w277) -> ()  [unwired: 2 in, 2 out]
                }
                frame #3 {
                  n285 = property on="In bubbler" class="Clust (strict)"() -> ("Value"=w284:T6)  [unwired: 2 in, 2 out]
                  n286 = Unbundle By Name(w284) -> ("Run"=w283:bool, "Prep"=w282:bool)
                  n287 = property on="Status Out" class="Str"() -> ("Value"=w290:string)  [unwired: 2 in, 2 out]
                  n288 = property on="first" class="Bool (strict)"() -> ("Value"=w288:bool)  [unwired: 2 in, 2 out]
                  n289 = call "flow_strings.vi"("string in"=w290, "is first in?"=w288, "name"="In", "run source?"=w283, "prep source?"=w282, "is prep?"=w285) -> ("string out"=w287:string, "is first out?"=w286:bool)  [unwired: 1 in]
                  n290 = property on="Status Out" class="Str"("Value"=w287) -> ()  [unwired: 2 in, 2 out]
                  n291 = property on="first" class="Bool (strict)"("Value"=w286) -> ()  [unwired: 2 in, 2 out]
                }
                frame #4 {
                  n292 = property on="P gas" class="Clust (strict)"() -> ("Value"=w293:T6)  [unwired: 2 in, 2 out]
                  n293 = Unbundle By Name(w293) -> ("Run"=w292:bool, "Prep"=w291:bool)
                  n294 = property on="Status Out" class="Str"() -> ("Value"=w298:string)  [unwired: 2 in, 2 out]
                  n295 = property on="first" class="Bool (strict)"() -> ("Value"=w296:bool)  [unwired: 2 in, 2 out]
                  n296 = call "flow_strings.vi"("string in"=w298, "is first in?"=w296, "name"="PH3", "run source?"=w292, "prep source?"=w291, "is prep?"=w294) -> ("string out"=w297:string, "is first out?"=w295:bool)  [unwired: 1 in]
                  n297 = property on="Status Out" class="Str"("Value"=w297) -> ()  [unwired: 2 in, 2 out]
                  n298 = property on="first" class="Bool (strict)"("Value"=w295) -> ()  [unwired: 2 in, 2 out]
                }
                frame #5 {
                  n299 = property on="As gas" class="Clust (strict)"() -> ("Value"=w302:T6)  [unwired: 2 in, 2 out]
                  n300 = Unbundle By Name(w302) -> ("Run"=w301:bool, "Prep"=w300:bool)
                  n301 = property on="Status Out" class="Str"() -> ("Value"=w307:string)  [unwired: 2 in, 2 out]
                  n302 = property on="first" class="Bool (strict)"() -> ("Value"=w305:bool)  [unwired: 2 in, 2 out]
                  n303 = call "flow_strings.vi"("string in"=w307, "is first in?"=w305, "name"="AsH3", "run source?"=w301, "prep source?"=w300, "is prep?"=w303) -> ("string out"=w304:string, "is first out?"=w306:bool)  [unwired: 1 in]
                  n304 = property on="Status Out" class="Str"("Value"=w304) -> ()  [unwired: 2 in, 2 out]
                  n305 = property on="first" class="Bool (strict)"("Value"=w306) -> ()  [unwired: 2 in, 2 out]
                }
                frame #6 {
                  n306 = property on="P bubbler" class="Clust (strict)"() -> ("Value"=w311:T6)  [unwired: 2 in, 2 out]
                  n307 = Unbundle By Name(w311) -> ("Run"=w310:bool, "Prep"=w309:bool)
                  n308 = property on="Status Out" class="Str"() -> ("Value"=w317:string)  [unwired: 2 in, 2 out]
                  n309 = property on="first" class="Bool (strict)"() -> ("Value"=w315:bool)  [unwired: 2 in, 2 out]
                  n310 = call "flow_strings.vi"("string in"=w317, "is first in?"=w315, "name"="P liq", "run source?"=w310, "prep source?"=w309, "is prep?"=w312) -> ("string out"=w314:string, "is first out?"=w313:bool)  [unwired: 1 in]
                  n311 = property on="Status Out" class="Str"("Value"=w314) -> ()  [unwired: 2 in, 2 out]
                  n312 = property on="first" class="Bool (strict)"("Value"=w313) -> ()  [unwired: 2 in, 2 out]
                }
                frame #7 {
                  n313 = property on="Zn bubbler" class="Clust (strict)"() -> ("Value"=w320:T7)  [unwired: 2 in, 2 out]
                  n314 = Unbundle By Name(w320) -> ("Bubbler (main).Run"=w319:bool, "Bubbler (main).Prep"=w318:bool)
                  n315 = property on="Status Out" class="Str"() -> ("Value"=w326:string)  [unwired: 2 in, 2 out]
                  n316 = property on="first" class="Bool (strict)"() -> ("Value"=w324:bool)  [unwired: 2 in, 2 out]
                  n317 = call "flow_strings.vi"("string in"=w326, "is first in?"=w324, "name"="Zn", "run source?"=w319, "prep source?"=w318, "is prep?"=w321) -> ("string out"=w323:string, "is first out?"=w322:bool)  [unwired: 1 in]
                  n318 = property on="Status Out" class="Str"("Value"=w323) -> ()  [unwired: 2 in, 2 out]
                  n319 = property on="first" class="Bool (strict)"("Value"=w322) -> ()  [unwired: 2 in, 2 out]
                }
                frame #8 {
                  n320 = property on="Se bubbler" class="Clust (strict)"() -> ("Value"=w329:T7)  [unwired: 2 in, 2 out]
                  n321 = Unbundle By Name(w329) -> ("Bubbler (main).Run"=w328:bool, "Bubbler (main).Prep"=w327:bool)
                  n322 = property on="Status Out" class="Str"() -> ("Value"=w335:string)  [unwired: 2 in, 2 out]
                  n323 = property on="first" class="Bool (strict)"() -> ("Value"=w333:bool)  [unwired: 2 in, 2 out]
                  n324 = call "flow_strings.vi"("string in"=w335, "is first in?"=w333, "name"="Se", "run source?"=w328, "prep source?"=w327, "is prep?"=w330) -> ("string out"=w332:string, "is first out?"=w331:bool)  [unwired: 1 in]
                  n325 = property on="Status Out" class="Str"("Value"=w332) -> ()  [unwired: 2 in, 2 out]
                  n326 = property on="first" class="Bool (strict)"("Value"=w331) -> ()  [unwired: 2 in, 2 out]
                }
              }
            }
            frame #3 {
              n327 = property on="run started" class="Bool (strict)"() -> ("Value"=w341:bool)  [unwired: 2 in, 2 out]
              n328 = Not(x=w341) -> (.not. x?=w340:bool)
              n329 = property on="prep_done" class="Bool (strict)"() -> ("Value"=w342:bool)  [unwired: 2 in, 2 out]
              n330 = And(x=w342, y=w340) -> (x .and. y?=w336:bool)
              n331 = case shown="False" w336 {
                selector: w336 -> [_ w344]
                tunnel: w339 -> [w343 w347]
                tunnel: [w343 w346] -> w338
                tunnel: w337 -> [_ w345]
                frame False {
                }
                frame True {
                  n332 = stacked-sequence {
                    tunnel: w345 -> [w349 _]
                    tunnel: w347 -> [_ w360]
                    tunnel: [_ w359] -> w346
                    tunnel: w344 -> [w348 _]
                    frame #0 {
                      n333 = case shown="True" w349 {
                        tunnel: w348 -> [w358 _]
                        frame False {
                          n334 = property on="Ga bubbler" class="Clust (strict)"() -> ("Value"=w356:T7)  [unwired: 2 in, 2 out]
                          n335 = property on="In bubbler" class="Clust (strict)"() -> ("Value"=w355:T6)  [unwired: 2 in, 2 out]
                          n336 = property on="P gas" class="Clust (strict)"() -> ("Value"=w354:T6)  [unwired: 2 in, 2 out]
                          n337 = property on="Al bubbler" class="Clust (strict)"() -> ("Value"=w357:T6)  [unwired: 2 in, 2 out]
                          n338 = property on="Zn bubbler" class="Clust (strict)"() -> ("Value"=w350:T7)  [unwired: 2 in, 2 out]
                          n339 = property on="Se bubbler" class="Clust (strict)"() -> ("Value"=w351:T7)  [unwired: 2 in, 2 out]
                          n340 = property on="As gas" class="Clust (strict)"() -> ("Value"=w353:T6)  [unwired: 2 in, 2 out]
                          n341 = property on="P bubbler" class="Clust (strict)"() -> ("Value"=w352:T6)  [unwired: 2 in, 2 out]
                          n342 = call "Set_V_III.vi"("Se bubbler"=w351, "P bubbler"=w352, "As gas"=w353, "P gas"=w354, "Run Started"=w358, "Zn bubbler"=w350, "In bubbler"=w355, "Ga bubbler"=w356, "Al bubbler"=w357) -> ()  [unwired: 3 in]
                        }
                        frame True {
                        }
                      }
                    }
                    frame #1 {
                      n343 = call "Set_Argument.vi"("Enable"=TRUE, "Argument"="run_started", "Argument List In"=w360) -> ("Argument List Out"=w359:string[])
                    }
                  }
                }
              }
            }
          }
        }
        frame "End" {
        }
        frame "Idle" {
        }
      }
    }
  }
  "Argument List Out" <- w10
  n344 = control-ref of="Ga bubbler"() -> ()  [unwired: 1 out]
